vi "Start.vi"   [LabVIEW 2019]
uses:
  <vilib>/rvi/eio/common/nirviEmuTemplateMethod_errors.vi
  <vilib>/eio/EIONode/EIONode.xnode
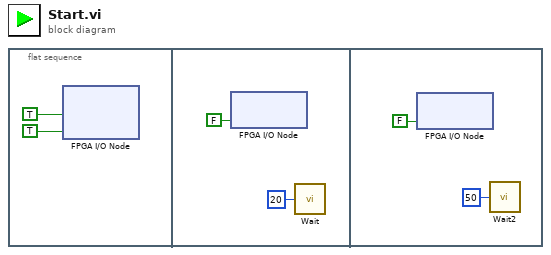
[diagram p0: block diagram]
diagram:
  n1 = flat-sequence {
    frame #0 {
      n2 = xnode "FPGA I/O Node"("SDA"=TRUE, "SCL"=TRUE) -> ()  [unwired: 2 in, 2 out]
    }
    frame #1 {
      n3 = xnode "FPGA I/O Node"("SDA"=FALSE) -> ()  [unwired: 1 in, 1 out]
      n4 = call "Wait"("Count(mSec)"=u32 20) -> ()  [unwired: 1 out]
    }
    frame #2 {
      n5 = xnode "FPGA I/O Node"("SCL"=FALSE ("SDA")) -> ()  [unwired: 1 in, 1 out]
      n6 = call "Wait2"("Count(mSec)"=u32 50) -> ()  [unwired: 1 out]
    }
  }
